vi "Spot Grid.vi"() -> ()   [LabVIEW 2016]
uses:
  <vilib>/imath/engines/lvmath2/RunTimeEngine/RangeToken/NIMS_Range.vi
  <instcachedir>/0/NIMS_Range_B290C9A4B417448F8AD7612DC5651788.lvgen/NIMS_Range_B290C9A4B417448F8AD7612DC5651788_001.vi
  <vilib>/imath/engines/lvmath2/RunTimeEngine/BuiltInFunctions/meshgrid2d/NIMS_meshgrid2d(V,V).vi
  <instcachedir>/0/NIMS_meshgrid2d(V,V)_3733343E1C554A708015CFB0432C6A59.lvgen/NIMS_meshgrid2d(V,V)_3733343E1C554A708015CFB0432C6A59_000.vi
  <vilib>/imath/engines/lvmath2/RunTimeEngine/ErrorHandling/NIMS_Create Error From Enums.vi
  <vilib>/imath/engines/lvmath2/RunTimeEngine/IndexRead/NIMS M($).vi
  <instcachedir>/0/NIMS M($)_82D1177398184AFB96A6AFB63C3C3F57.lvgen/NIMS M($)_82D1177398184AFB96A6AFB63C3C3F57_000.vi
  <vilib>/imathl/engines/lvmath/Functions/Error Handling/Create Error.vi
  <vilib>/imath/engines/lvmath2/RunTimeEngine/BuiltInFunctions/length/NIMS_length(GV).vi
  <instcachedir>/0/NIMS_length(GV)_08A3D13377FD4E4B96F5795FBF3698FA.lvgen/NIMS_length(GV)_08A3D13377FD4E4B96F5795FBF3698FA_000.vi
  <vilib>/imath/engines/lvmath2/RunTimeEngine/BuiltInFunctions/zeros/NIMS_V=zeros(I32,I32).vi
  <vilib>/imath/engines/lvmath2/RunTimeEngine/BuiltInFunctions/ones/NIMS_V=ones(I32,I32).vi
  <vilib>/imath/engines/lvmath2/RunTimeEngine/NodeEndStatement/NIMS_NodeEndStatement_Output.vi
  <instcachedir>/0/NIMS_NodeEndStatement_Output_53EC0D466D134D7ABD903AC30B43404B.lvgen/NIMS_NodeEndStatement_Output_53EC0D466D134D7ABD903AC30B43404B_005.vi
  <vilib>/imath/engines/lvmath2/RunTimeEngine/ErrorHandling/NIMS_Finalize Error.vi
panel:
  out "z_spots":dbl[](array[numeric])
  out "I_spots":dbl[](array[numeric])
  in  "I0":dbl=1.0
  in  "x0":i32
  in  "y0":i32
  in  "dx":i32=32
  in  "dy":i32=32
  in  "ny":i32=5
  in  "ny":i32=5
  out "XY Graph":cluster{"X":dbl[], "Y":dbl[]}(graph)
  out "y_spots":dbl[](array[numeric])
  out "x_spots":dbl[](array[numeric])
  in  "Stop":bool
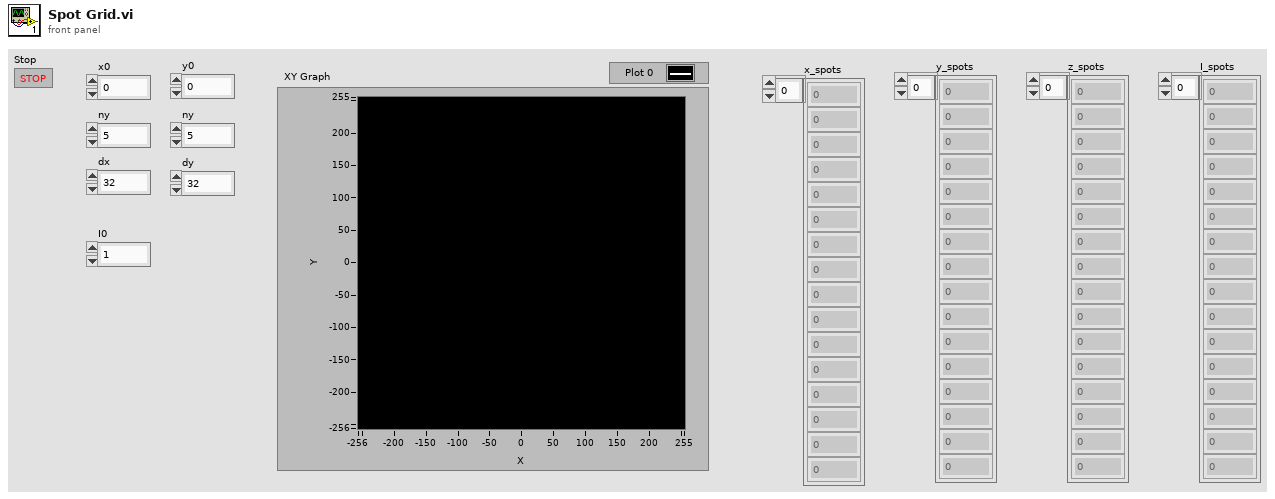
[diagram p1: front panel]
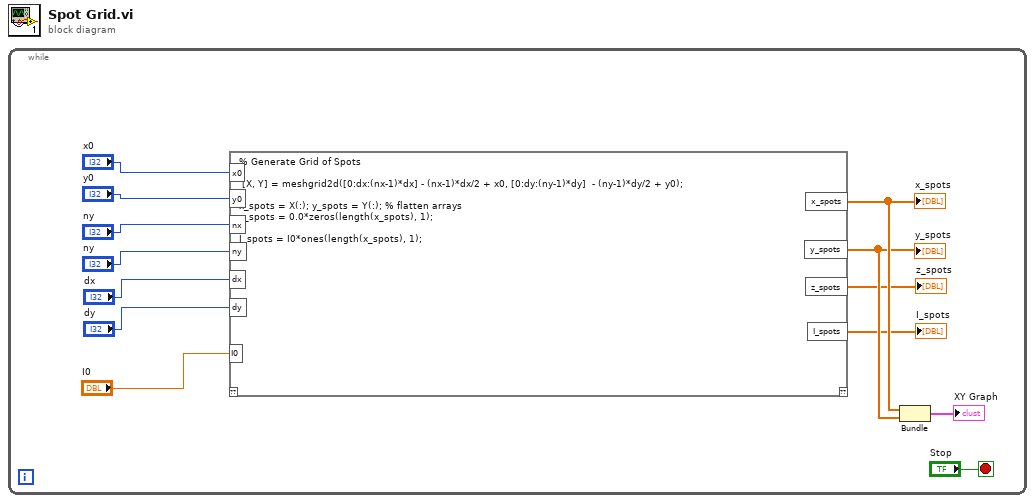
[diagram p0: block diagram]
diagram:
  n1 = while {
    stop <- "Stop" stop-if-true
    n2 = mathscript code="% Generate Grid of Spots\n\n [X, Y] = meshgrid2d([0:dx:(nx-1)*dx] - (nx-1)*dx/2 + x0, [0:dy:(ny-1)*dy]  - (ny-1)*dy/2 + y0);\n\nx_spots = X(:); y_spots = Y(:); % flatten arrays\nz_spots = 0.0*zeros(length(x_spots), 1);\n\nI_spots = I0*ones(length(x_spots), 1);"("nx"="ny", "ny"="ny", "dx"="dx", "dy"="dy", "x0"="x0", "y0"="y0", "I0"="I0") -> ("x_spots"=w12:dbl[], "y_spots"=w10:dbl[], "I_spots"=→"I_spots":dbl[], "z_spots"=→"z_spots":dbl[])  [unwired: 1 in, 1 out]
    "x_spots" <- w12
    "y_spots" <- w10
    n3 = Bundle("x_spots"=w12, "y_spots"=w10) -> (→"XY Graph":cluster{"x_spots":dbl[], "y_spots":dbl[]})  [unwired: 1 in]
  }
